vi "openPathInExplorer.vi"(8 "error in (no error)":errorcluster, 11 "pathToOpen":path) -> (0 "error out":errorcluster)   [LabVIEW 2023]
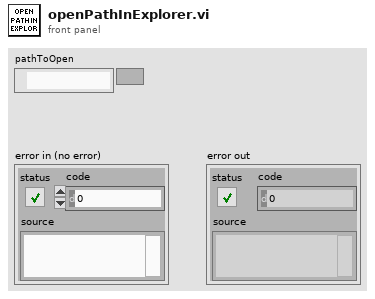
[diagram p1: front panel]
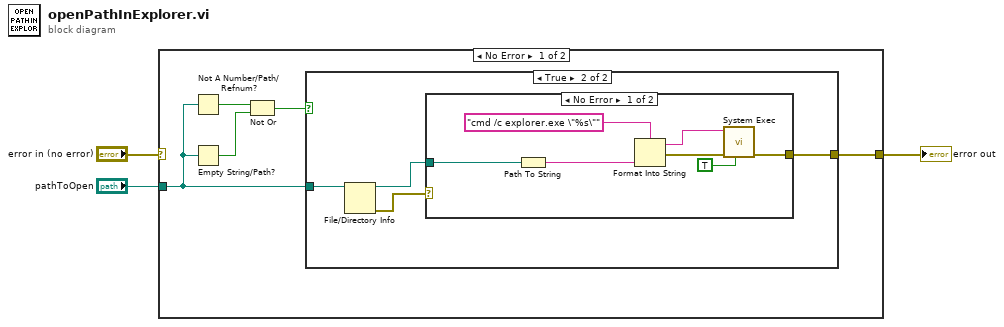
[diagram p0: block diagram]
diagram:
  n1 = case shown="No Error" "error in (no error)" {
    selector: "error in (no error)" -> [_ w20]
    tunnel: "pathToOpen" -> [w8 _]
    tunnel: [w4 w20] -> w1
    frame No Error {
      n2 = Not A Number/Path/Refnum?(number/path/refnum=w8) -> (NaN/Path/Refnum?=w6:bool)
      n3 = Empty String/Path?(string/path=w8) -> (empty?=w5:bool)
      n4 = Not Or(1:w5, 2:w6) -> (0:w7:bool)
      n5 = case shown="True" w7 {
        tunnel: w8 -> [_ w11]
        tunnel: [_ w9] -> w4
        frame False {
        }
        frame True {
          n6 = File/Directory Info(path=w11) -> (path out=w10:path, error out=w12:errorcluster)  [unwired: 1 in, 5 out]
          n7 = case shown="No Error" w12 {
            tunnel: w10 -> [w14 _]
            tunnel: [w13 _] -> w9
            frame No Error {
              n8 = Path To String(path=w14) -> (string=w19:string)
              n9 = Format Into String(format string="cmd /c explorer.exe \"%s\"", w19) -> (resulting string=w17:string, error out=w16:errorcluster)  [unwired: 2 in]
              n10 = call <vilib>:"System Exec.vi"("run minimized? (F)"=TRUE, "error in (no error)"=w16, "command line"=w17) -> ("error out"=w13:errorcluster)  [unwired: 5 in, 3 out]
            }
            frame Error {
            }
          }
        }
      }
    }
    frame Error {
    }
  }
  "error out" <- w1
